vi "Init FD.vi"(8 "error in":errorcluster, 9 "BitrateFD":string, 10 "Channel":T2=81 items=["PCAN_NONEBUS"=0, "PCAN_USBBUS1"=81, "PCAN_USBBUS2"=82, "PCAN_USBBUS3"=83, "PCAN_USBBUS4"=84, "PCAN_USBBUS5"=85, "PCAN_USBBUS6"=86, "PCAN_USBBUS7"=87, "PCAN_USBBUS8"=88, "PCAN_USBBUS9"=1289, "PCAN_USBBUS10"=1290, "PCAN_USBBUS11"=1291, "PCAN_USBBUS12"=1292, "PCAN_USBBUS13"=1293, "PCAN_USBBUS14"=1294, "PCAN_USBBUS15"=1295, "PCAN_USBBUS16"=1296]) -> (0 "error out":errorcluster, 3 "TPCANHandle out":T2=81 items=["PCAN_NONEBUS"=0, "PCAN_USBBUS1"=81, "PCAN_USBBUS2"=82, "PCAN_USBBUS3"=83, "PCAN_USBBUS4"=84, "PCAN_USBBUS5"=85, "PCAN_USBBUS6"=86, "PCAN_USBBUS7"=87, "PCAN_USBBUS8"=88, "PCAN_USBBUS9"=1289, "PCAN_USBBUS10"=1290, "PCAN_USBBUS11"=1291, "PCAN_USBBUS12"=1292, "PCAN_USBBUS13"=1293, "PCAN_USBBUS14"=1294, "PCAN_USBBUS15"=1295, "PCAN_USBBUS16"=1296], 5 "TPCANStatus":T1 items=["PCAN_ERROR_OK"=0, "PCAN_ERROR_XMTFULL"=1, "PCAN_ERROR_OVERRUN"=2, "PCAN_ERROR_BUSLIGHT"=4, "PCAN_ERROR_BUSHEAVY"=8, "PCAN_ERROR_BUSPASSIVE"=262144, "PCAN_ERROR_BUSOFF"=16, "PCAN_ERROR_QRCVEMPTY"=32, "PCAN_ERROR_QOVERRUN"=64, "PCAN_ERROR_QXMTFULL"=128, "PCAN_ERROR_REGTEST"=256, "PCAN_ERROR_NODRIVER"=512, "PCAN_ERROR_HWINUSE"=1024, "PCAN_ERROR_NETINUSE"=2048, "PCAN_ERROR_ILLHW"=5120, "PCAN_ERROR_ILLNET"=6144, "PCAN_ERROR_ILLCLIENT"=7168, "PCAN_ERROR_RESOURCE"=8192, "PCAN_ERROR_ILLPARAMTYPE"=16384, "PCAN_ERROR_ILLPARAMVAL"=32768, "PCAN_ERROR_UNKNOWN"=65536, "PCAN_ERROR_ILLDATA"=131072, "PCAN_ERROR_ILLMODE"=524288, "PCAN_ERROR_CAUTION"=33554432, "PCAN_ERROR_INITIALIZE"=67108864, "PCAN_ERROR_ILLOPERATION"=134217728])   [LabVIEW 2018, in "PCANBasic.lvlib"]
doc: "Initializes a FD capable PCAN Channel \n\nAs indicated by its name, the Initialize method initiates a PCAN Channel, preparing it for communicate within the CAN bus connected to it. Calls to the other methods will fail if they are used with a Channel handle, different than PCAN_NONEBUS, that has not been initialized yet. Each initialized channel should be released when it is not needed anymore. \n\nInitializing a PCAN Channel means:\n\nto reserve the Channel for the calling application/process. \nto allocate channel resources, like receive and transmit queues. \nto register/connect the Hardware denoted by the channel handle. \nto check and adapt the bus speed, if the Channel is already in use. (Only if the Channel was pre-configured as Bitrate Adapting; see: Bitrate-Adapting Parameter). \nto set the channel in Listen-Only mode. (Only if the channel was pre-configured as Listen-Only; see: Listen-Only Parameter). \nto open the messages filter for the application/process. \nto set-up the default values of the different parameters (See GetValue). \nto set the Receive Status of the channel. (Pre-configured value; see: Receive Status Parameter). \nWhat is different from the PCAN-Light API, the Initialization process will fail if an application tries to initialize a PCAN-Channel that has been initialized already within the same process. \n\nTake in consideration that initializing a channel causes a reset of the CAN hardware , when the bus status is other than OK. In this way errors like BUSOFF, BUSHEAVY, and BUSLIGHT, are removed."
uses:
  PCANBasic.lvlib
  TPCANHandle.ctl
  TPCANStatus.ctl
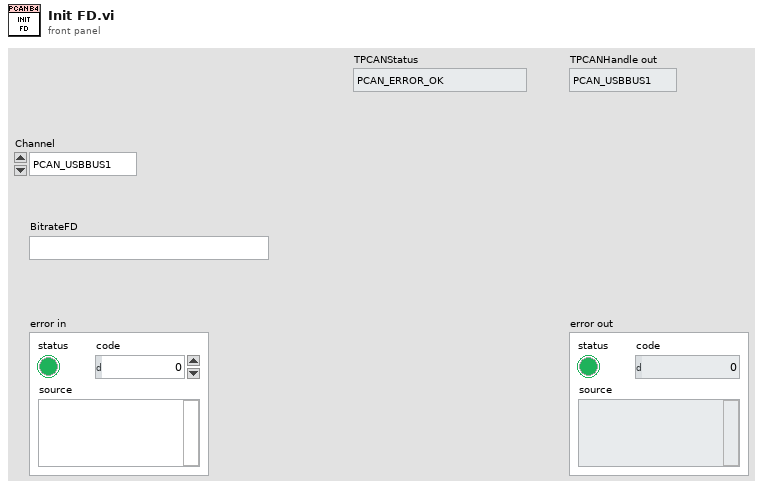
[diagram p1: front panel]
types:
  T1 = typedef "PCANBasic.lvlib/TPCANStatus.ctl" = u32
  T2 = typedef "PCANBasic.lvlib/TPCANHandle.ctl" = u16
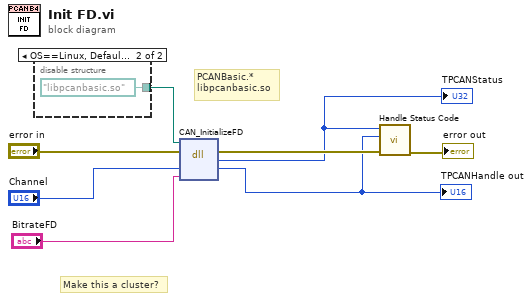
[diagram p0: block diagram]
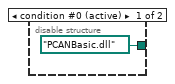
[diagram p2: hidden frame]
diagram:
  # "Make this a cluster?"
  # "PCANBasic.*\nlibpcanbasic.so"
  n1 = disable-structure shown="OS==Linux, Default" {
    disable-tunnel: [path "PCANBasic.dll" path "libpcanbasic.so"] -> w5
    frame condition #0 (active) {
    }
    frame condition #1 {
    }
  }
  n2 = dll-call lib="?" fn="CAN_InitializeFD"(path in=w5, error in="error in", "Channel"="Channel", "BitrateFD"="BitrateFD") -> (error out=w7:errorcluster, "TPCANStatus"=w3:u32, "Channel"=w2:u16)  [unwired: 2 in, 1 out]
  "TPCANHandle out" <- w2
  "TPCANStatus" <- w3
  n3 = call "Handle Status Code.vi"("error in"=w7, "TPCANHandle"=w2, "TPCANStatus"=w3) -> ("error out"=→"error out":errorcluster)  [unwired: 8 in]
